vi "Eagle_FPGA Scanner Control_2.vi"() -> ()   [LabVIEW 2015]
uses:
  <vilib>/rvi/Emulation/niFpgaGetClockAttributes.vi
  <vilib>/rvi/Emulation/niFpgaSctlEmulationGetInTimedLoop.vi
  <vilib>/rvi/Emulation/niFpgaEmulationReportErrorSimple.vi
  <vilib>/rvi/eio/common/nirviEmuTemplateMethod_errors.vi
  <vilib>/rvi/Emulation/niFpgaCriticalErrorInLSC.vi
  <vilib>/rvi/FXPMathLib/FxpMul/XNode/nifxpmath_Multiplier.xnode
  <vilib>/eio/EIONode/EIONode.xnode
  <vilib>/rvi/FXPMathLib/sim/FxpSim.dll
  <vilib>/rvi/FXPMathLib/FxpAdd/XNode/nifxpmath_Add.xnode
panel:
  out "-Y CMD IND":fxp<+/-,20,5>
  out "-X CMD IND":fxp<+/-,20,5>
  in  "VY":fxp<+/-,20,5>
  in  "VX":fxp<+/-,20,5>
  out "Y CMD IND":fxp<+/-,20,5>
  out "X CMD IND":fxp<+/-,20,5>
  out "Mod3/AI1":fxp<+,18,3>
  out "Mod3/AI0":fxp<+,18,3>
  in  "Mod3/AO1":fxp<+,16,3>
  in  "Mod3/AO0":fxp<+,16,3>
  out "Y READ":fxp<+/-,20,5>
  out "X READ":fxp<+/-,20,5>
  in  "Y":fxp<+,20,10>
  in  "Y MULT":fxp<+/-,20,5>
  in  "Y OFFS":fxp<+/-,20,5>
  in  "X OFFS":fxp<+/-,20,5>
  in  "X MULT":fxp<+/-,20,5>
  in  "X":fxp<+,20,10>
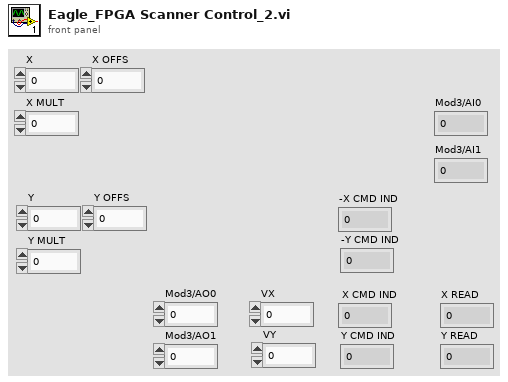
[diagram p1: front panel]
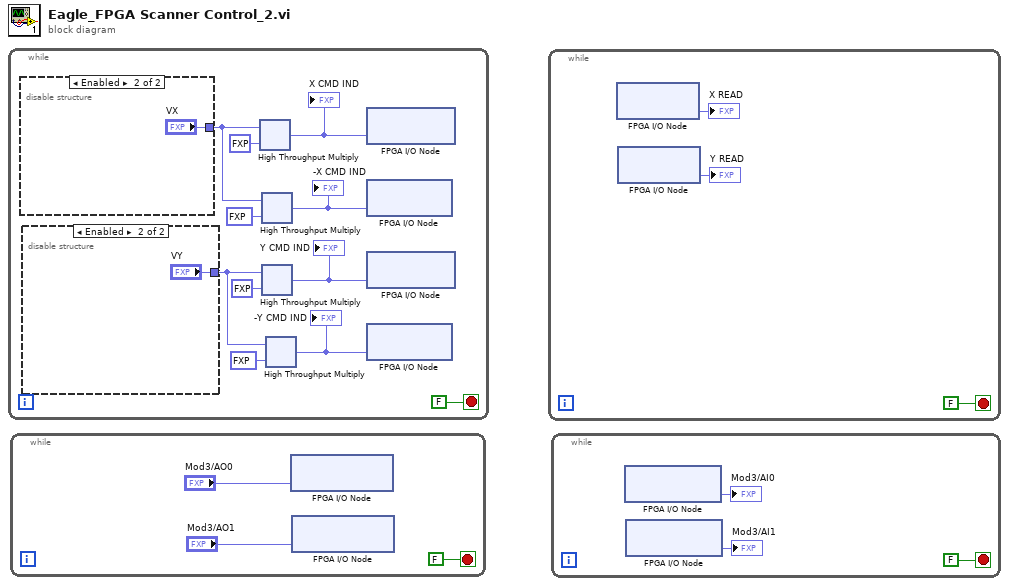
[diagram p0: block diagram]
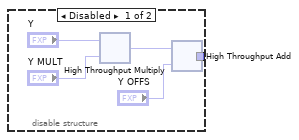
[diagram p2: hidden frame]
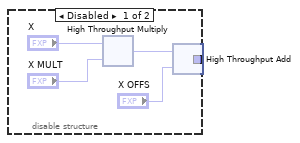
[diagram p3: hidden frame]
diagram:
  n1 = while {
    stop <- FALSE stop-if-true
    n2 = disable-structure shown="Enabled" {
      disable-tunnel: [w18 "VX"] -> w5
      frame Disabled {
        n3 = xnode ("High Throughput Multiply")("x"="X", "y"="X MULT") -> ("x*y"=w22:fxp<+/-,40,15>)
        n4 = xnode ("High Throughput Add")("x"=w22, "y"="X OFFS") -> ("x+y"=w18:fxp<+/-,41,16>)
      }
      frame Enabled {
      }
    }
    n5 = disable-structure shown="Enabled" {
      disable-tunnel: [w12 "VY"] -> w1
      frame Disabled {
        n6 = xnode ("High Throughput Multiply")("x"="Y", "y"="Y MULT") -> ("x*y"=w13:fxp<+/-,40,15>)
        n7 = xnode ("High Throughput Add")("x"=w13, "y"="Y OFFS") -> ("x+y"=w12:fxp<+/-,41,16>)
      }
      frame Enabled {
      }
    }
    n8 = xnode ("High Throughput Multiply")("x"=w5, "y"=fxp<+/-,20,5> 0.5) -> ("x*y"=w8:fxp<+/-,20,5>)
    "X CMD IND" <- w8
    n9 = xnode ("High Throughput Multiply")("x"=w5, "y"=fxp<+/-,20,5> -0.5) -> ("x*y"=w6:fxp<+/-,20,5>)
    "-X CMD IND" <- w6
    n10 = xnode ("High Throughput Multiply")("x"=w1, "y"=fxp<+/-,20,5> 0.5) -> ("x*y"=w3:fxp<+/-,20,5>)
    "Y CMD IND" <- w3
    n11 = xnode ("High Throughput Multiply")("x"=w1, "y"=fxp<+/-,20,5> -0.5) -> ("x*y"=w2:fxp<+/-,20,5>)
    "-Y CMD IND" <- w2
    n12 = xnode "FPGA I/O Node"("X CMD+"=w8) -> ()  [unwired: 1 in, 1 out]
    n13 = xnode "FPGA I/O Node"("X CMD-"=w6) -> ()  [unwired: 1 in, 1 out]
    n14 = xnode "FPGA I/O Node"("Y CMD+"=w3) -> ()  [unwired: 1 in, 1 out]
    n15 = xnode "FPGA I/O Node"("Y CMD-"=w2) -> ()  [unwired: 1 in, 1 out]
  }
  n16 = while {
    stop <- FALSE stop-if-true
    n17 = xnode "FPGA I/O Node"("Mod3/AO0"="Mod3/AO0") -> ()  [unwired: 1 in, 1 out]
    n18 = xnode "FPGA I/O Node"("Mod3/AO1"="Mod3/AO1") -> ()  [unwired: 1 in, 1 out]
  }
  n19 = while {
    stop <- FALSE stop-if-true
    n20 = xnode "FPGA I/O Node"() -> ("X READ"=→"X READ":fxp<+/-,20,5>)  [unwired: 1 in, 1 out]
    n21 = xnode "FPGA I/O Node"() -> ("Y READ"=→"Y READ":fxp<+/-,20,5>)  [unwired: 1 in, 1 out]
  }
  n22 = while {
    stop <- FALSE stop-if-true
    n23 = xnode "FPGA I/O Node"() -> ("Mod3/AI0"=→"Mod3/AI0":fxp<+,18,3>)  [unwired: 1 in, 1 out]
    n24 = xnode "FPGA I/O Node"() -> ("Mod3/AI1"=→"Mod3/AI1":fxp<+,18,3>)  [unwired: 1 in, 1 out]
  }
